vi "Generate_WayPoints_Hopping WITH Variable Retract Rates.vi"(8 "Update Position Loop Wait Time (us)":u32=50000, 11 "Input Cluster":T2={"Scan Rate (um/s)"=15.0, "X Start"=15.0, "X End"=15.0, "Y Start"=15.0, "Y End"=15.0, " Z Start"=15.0, "HoppingDistance"=1.0, "V"=15.0, "Z End"=15.0, "Approach Rate Hopping (um/s)"=15.0, "Retrack Rate (um/s)"=15.0, "V 2"=15.0, "Approach Rate (um/s)"=15.0, "Hold Time START / s"=15.0, "Hold Time Delta / s"=15.0}) -> (0 "output cluster":T1)   [LabVIEW 2023]
uses:
  TypeDefs/WayPointCluster.ctl
  User_Vi/Settings.vi
panel:
  in  "WayPointCluster":T1
  out "Y  P":dbl
  out "X  P":dbl
  out "HoppingDistanceX":dbl
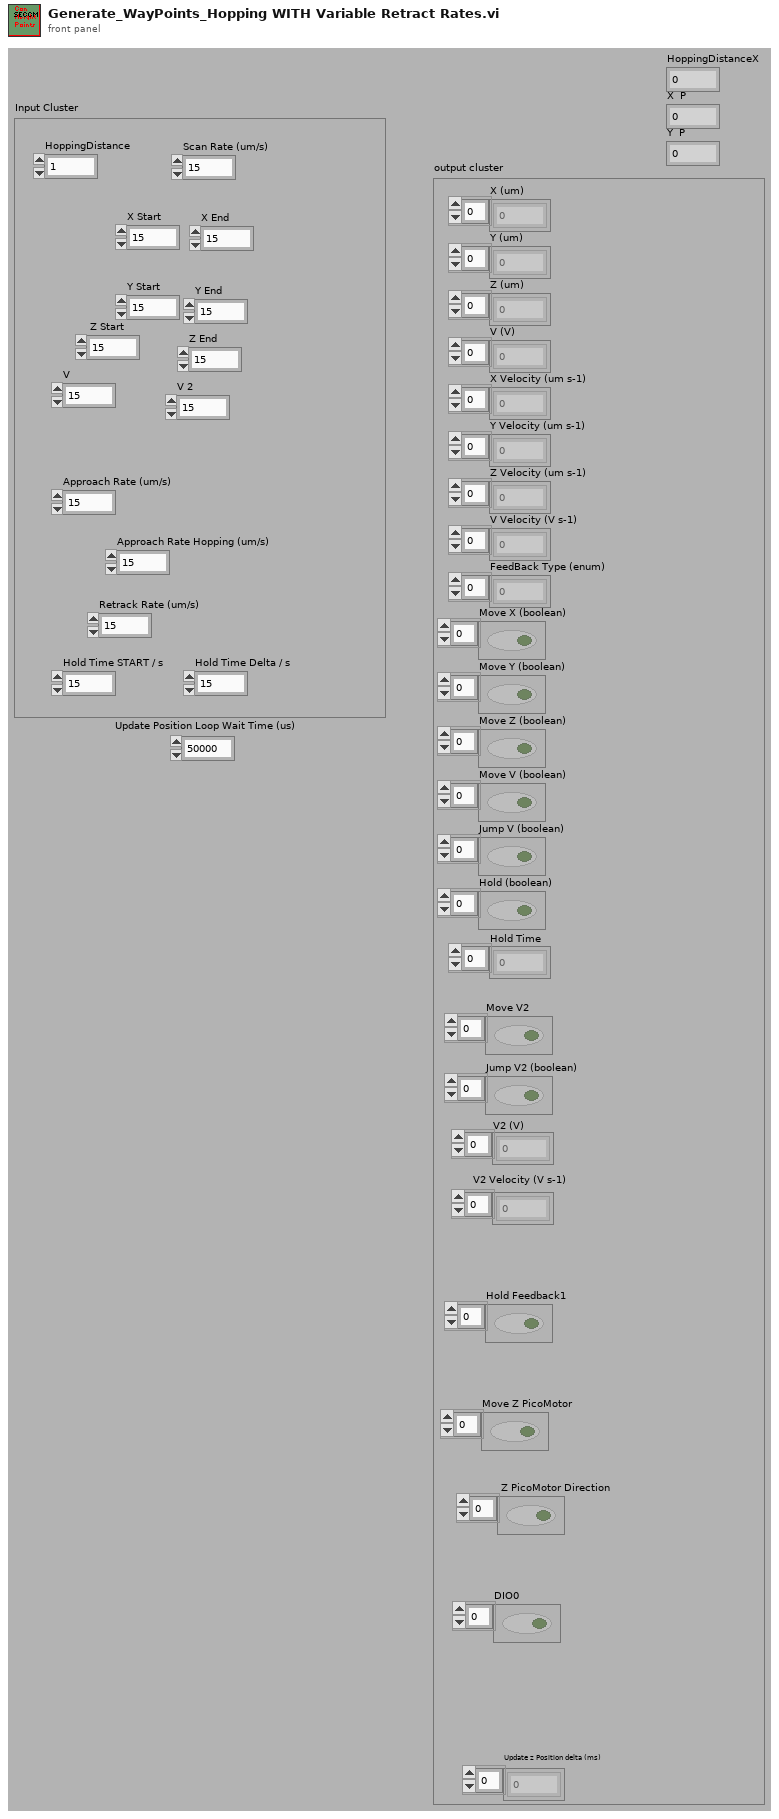
[diagram p1: front panel]
types:
  T1 = typedef "WayPointCluster.ctl" = cluster{"X (um)":dbl[], "Y (um)":dbl[], "Z (um)":dbl[], "V (V)":dbl[], "X Velocity (um s-1)":dbl[], "Y Velocity (um s-1)":dbl[], "Z Velocity (um s-1)":dbl[], "V Velocity (V s-1)":dbl[], "FeedBack Type (enum)":u16[], "Move X (boolean)":bool[], "Move Y (boolean)":bool[], "Move Z (boolean)":bool[], "Move V (boolean)":bool[], "Jump V (boolean)":bool[], "Hold (boolean)":bool[], "Hold Time":u32[], "V2 (V)":dbl[], "Move V2":bool[], "V2 Velocity (V s-1)":dbl[], "Jump V2 (boolean)":bool[], "Update z Position delta (ms)":i16[], "Hold Feedback1":bool[], "Move Z PicoMotor":bool[], " Z PicoMotor Direction":bool[], "DIO0":bool[]}
  T2 = cluster{"Scan Rate (um/s)":dbl, "X Start":dbl, "X End":dbl, "Y Start":dbl, "Y End":dbl, " Z Start":dbl, "HoppingDistance":dbl, "V":dbl, "Z End":dbl, "Approach Rate Hopping (um/s)":dbl, "Retrack Rate (um/s)":dbl, "V 2":dbl, "Approach Rate (um/s)":dbl, "Hold Time START / s":dbl, "Hold Time Delta / s":dbl}
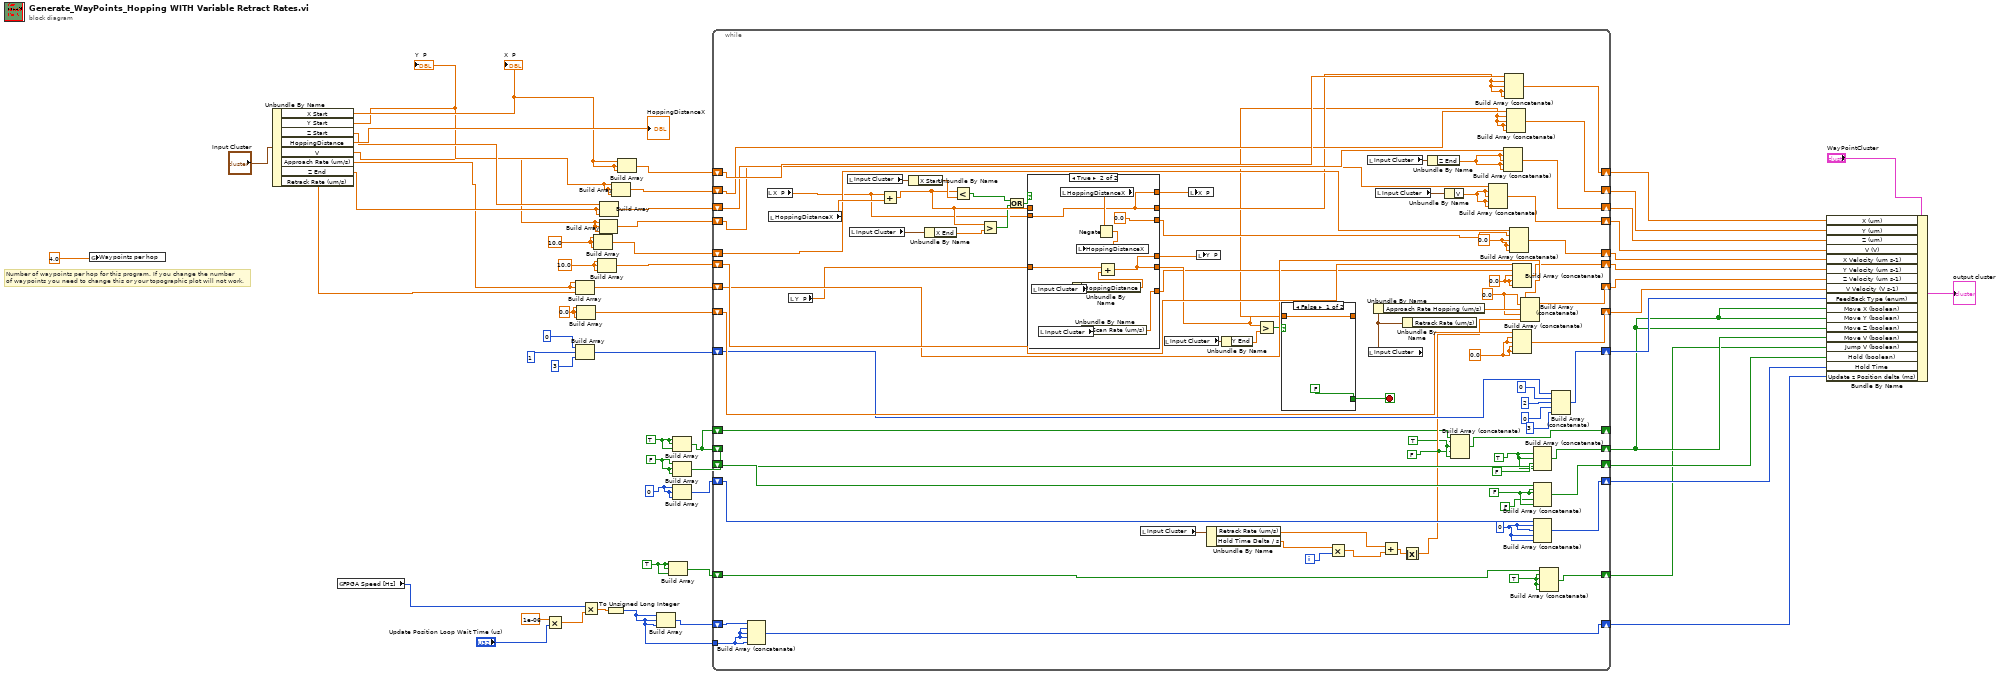
[diagram p0: block diagram]
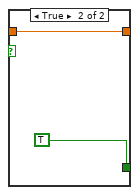
[diagram p2: hidden frame]
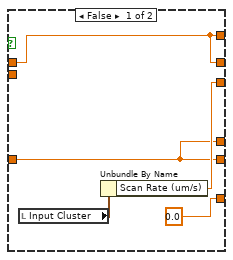
[diagram p3: hidden frame]
diagram:
  w20 = TRUE
  w19 = u32 0 ("element")
  w18 = FALSE
  w17 = TRUE
  w13 = 10.0 ("element")
  w14 = 10.0 ("element")
  w16 = 0.0 ("element")
  # "Number of waypoints per hop for this program. If you change the number\nof waypoints you need to change this or your topographic plot will not work."
  n1 = global write "Settings.vi" "Waypoints per hop"(4.0) -> ()
  n2 = Unbundle By Name("Input Cluster") -> ("X Start"=w35:dbl, "Y Start"=w34:dbl, "Z Start"=w36:dbl, "HoppingDistance"=→"HoppingDistanceX":dbl, "V"=w32:dbl, "Approach Rate (um/s)"=w15:dbl, "Z End"=w33:dbl, "Retrack Rate (um/s)"=w31:dbl)
  "X  P" <- w35
  "Y  P" <- w34
  n3 = global read "Settings.vi" "FPGA Speed [Hz]"() -> (w1:i64)
  n4 = Multiply(x=1e-06, y="Update Position Loop Wait Time (us)") -> (x*y=w10:dbl)
  n5 = Build Array(w15, w15, w31) -> (w43:dbl[])
  n6 = Build Array(u16 0 ("element"), u16 1 ("element"), u16 3 ("element")) -> (w39:u16[])
  n7 = Build Array(w16, w16, w16) -> (w41:dbl[])
  n8 = Multiply(x=w1, y=w10) -> (x*y=w5:dbl)
  n9 = Build Array(w13, w13, w13) -> (w46:dbl[])
  n10 = Build Array(w14, w14, w14) -> (w45:dbl[])
  n11 = Build Array(w32, w32, w32) -> (w48:dbl[])
  n12 = Build Array(w36, w33, w33) -> (w50:dbl[])
  n13 = To Unsigned Long Integer(number=w5) -> (unsigned 32bit integer=w4:u32)
  n14 = Build Array(w34, w34, w34) -> (w52:dbl[])
  n15 = Build Array(w35, w35, w35) -> (w54:dbl[])
  n16 = Build Array(w4, w4, w4) -> (w7:u32[])
  n17 = Build Array(w20, w20, w20) -> (w23:bool[])
  n18 = Build Array(w17, w17, w17) -> (w3:bool[])
  n19 = Build Array(w18, w18, w18) -> (w28:bool[])
  n20 = Build Array(w19, w19, w19) -> (w27:u32[])
  n21 = while {
    shift-right: [w134] -> w53
    shift-left: w54 -> [w135]
    shift-right: [w126] -> w51
    shift-left: w52 -> [w116]
    shift-right: [w125] -> w49
    shift-left: w50 -> [w133]
    shift-right: [w124] -> w47
    shift-left: w48 -> [w132]
    shift-right: [w123] -> w29
    shift-left: w46 -> [w131]
    shift-right: [w122] -> w44
    shift-left: w45 -> [w130]
    shift-right: [w121] -> w42
    shift-left: w43 -> [w129]
    shift-right: [w120] -> w40
    shift-left: w41 -> [w128]
    shift-right: [w119] -> w38
    shift-left: w39 -> [w127]
    shift-right: [w76] -> w26
    shift-left: w3 -> [w75]
    shift-right: [w77] -> w25
    shift-left: w28 -> [w84]
    shift-right: [w78] -> w24
    shift-left: w27 -> [w83]
    shift-right: [w72] -> w22
    shift-left: w23 -> [w73]
    shift-right: [w61] -> w6
    shift-left: w7 -> [w63]
    tunnel: w4 -> [w62]
    shift-right: [w58] -> _
    shift-left: w3 -> [w57]
    i -> [w69]
    stop <- w106 stop-if-true
    w59 = FALSE
    w60 = TRUE
    w71 = TRUE
    w68 = u32 0 ("element")
    w81 = FALSE
    w74 = TRUE
    w89 = 0.0 ("element")
    w90 = 0.0 ("element")
    w87 = 0.0 ("element")
    w88 = 0.0 ("element")
    n22 = Build Array (concatenate)(w63, w62, w62, w62, w62) -> (w61:u32[])
    n23 = local read "X  P"() -> (w104:dbl)
    n24 = local read "HoppingDistanceX"() -> (w136:dbl)
    n25 = local read "Y  P"() -> (w103:dbl)
    n26 = local read "Input Cluster"() -> (w138:T2)
    n27 = local read "Input Cluster"() -> (w137:T2)
    n28 = Add(x=w104, y=w136) -> (x+y=w112:dbl)
    n29 = Unbundle By Name(w138) -> ("X Start"=w115:dbl)
    n30 = Unbundle By Name(w137) -> ("X End"=w113:dbl)
    n31 = Less?(x=w112, y=w115) -> (x < y?=w114:bool)
    n32 = Greater?(x=w112, y=w113) -> (0:w111:bool)
    n33 = Or(x=w114, y=w111) -> (x .or. y?=w110:bool)
    n34 = case shown="True" w110 {
      tunnel: w112 -> [w143 _]
      tunnel: [w143 w149] -> w94
      tunnel: w104 -> [_ w149]
      tunnel: w103 -> [w144 w150]
      tunnel: [w144 w148] -> w102
      tunnel: [w146 0.0] -> w96
      tunnel: [0.0 w151] -> w95
      tunnel: [w144 w148] -> w101
      tunnel: [w143 w149] -> w100
      frame False {
        n35 = local read "Input Cluster"() -> (w147:T2)
        n36 = Unbundle By Name(w147) -> ("Scan Rate (um/s)"=w146:dbl)
      }
      frame True {
        n37 = local read "Input Cluster"() -> (w155:T2)
        n38 = local read "Input Cluster"() -> (w153:T2)
        n39 = local read "HoppingDistanceX"() -> (w157:dbl)
        n40 = Unbundle By Name(w155) -> ("HoppingDistance"=w154:dbl)
        n41 = Unbundle By Name(w153) -> ("Scan Rate (um/s)"=w151:dbl)
        n42 = Negate(x=w157) -> (-x=w156:dbl)
        n43 = local write "HoppingDistanceX"(w156) -> ()
        n44 = Add(x=w150, y=w154) -> (x+y=w148:dbl)
      }
    }
    n45 = local read "Input Cluster"() -> (w79:T2)
    n46 = local read "Input Cluster"() -> (w109:T2)
    n47 = local write "X  P"(w100) -> ()
    n48 = local write "Y  P"(w101) -> ()
    n49 = Unbundle By Name(w79) -> ("Retrack Rate (um/s)"=w64:dbl, "Hold Time Delta / s"=w70:dbl)
    n50 = Unbundle By Name(w109) -> ("Y End"=w108:dbl)
    n51 = Greater?(x=w102, y=w108) -> (0:w107:bool)
    n52 = case shown="False" w107 {
      tunnel: w102 -> [w140 w142]
      tunnel: [w140 w142] -> w93
      tunnel: [FALSE TRUE] -> w106
      frame False {
      }
      frame True {
      }
    }
    n53 = Multiply(x=w70, y=w69) -> (x*y=w65:dbl)
    n54 = local read "Input Cluster"() -> (w118:T2)
    n55 = local read "Input Cluster"() -> (w105:T2)
    n56 = Unbundle By Name(w105) -> ("Approach Rate Hopping (um/s)"=w97:dbl)
    n57 = local read "Input Cluster"() -> (w117:T2)
    n58 = Add(x=w64, y=w65) -> (x+y=w66:dbl)
    n59 = Unbundle By Name(w105) -> ()  [unwired: 1 out]
    n60 = Absolute Value(x=w66) -> (abs(x)=w67:dbl)
    n61 = Unbundle By Name(w118) -> ("Z End"=w92:dbl)
    n62 = Unbundle By Name(w117) -> ("V"=w91:dbl)
    n63 = Build Array (concatenate)(w57, w59, w60, w59, w60) -> (w58:bool[])
    n64 = Build Array (concatenate)(w132, w91, w91, w91, w91) -> (w124:dbl[])
    n65 = Build Array (concatenate)(w133, w92, w92, w92, w92) -> (w125:dbl[])
    n66 = Build Array (concatenate)(w135, w94, w94, w94, w94) -> (w134:dbl[])
    n67 = Build Array (concatenate)(w116, w93, w93, w93, w93) -> (w126:dbl[])
    n68 = Build Array (concatenate)(w131, w96, w90, w90, w90) -> (w123:dbl[])
    n69 = Build Array (concatenate)(w130, w95, w89, w89, w89) -> (w122:dbl[])
    n70 = Build Array (concatenate)(w128, w87, w87, w87, w87) -> (w120:dbl[])
    n71 = Build Array (concatenate)(w129, w88, w97, w88, w67) -> (w121:dbl[])
    n72 = Build Array (concatenate)(w75, w74, w74, FALSE, w74) -> (w76:bool[])
    n73 = Build Array (concatenate)(w84, w81, w81, FALSE, w81) -> (w77:bool[])
    n74 = Build Array (concatenate)(w83, w68, w68, w68, w68) -> (w78:u32[])
    n75 = Build Array (concatenate)(w73, w71, w71, w71, w71) -> (w72:bool[])
    n76 = Build Array (concatenate)(w127, u16 0 ("element"), u16 2 ("element"), u16 0 ("element"), u16 3 ("element")) -> (w119:u16[])
  }
  n77 = Bundle By Name(cluster="WayPointCluster", "X (um)"=w53, "Y (um)"=w51, "Z (um)"=w49, "V (V)"=w47, "X Velocity (um s-1)"=w29, "Y Velocity (um s-1)"=w44, "Z Velocity (um s-1)"=w42, "V Velocity (V s-1)"=w40, "FeedBack Type (enum)"=w38, "Move X (boolean)"=w26, "Move Y (boolean)"=w26, "Move Z (boolean)"=w26, "Move V (boolean)"=w26, "Jump V (boolean)"=w22, "Hold (boolean)"=w25, "Hold Time"=w24, "Update z Position delta (ms)"=w6) -> (→"output cluster":T1)
